vi "Parse Opening Tag.vi"(8 "Error In":errorcluster, 11 "Parser In":refnum<class "Parser.lvclass">) -> (0 "Error Out":errorcluster, 3 "Parser Out":refnum<class "Parser.lvclass">)   [LabVIEW 2017, in "Mustache.lvlib" / "Parser.lvclass"]
uses:
  Parser.lvclass
  Parser.lvclass/Parser.ctl
  Public/Controls/States.ctl
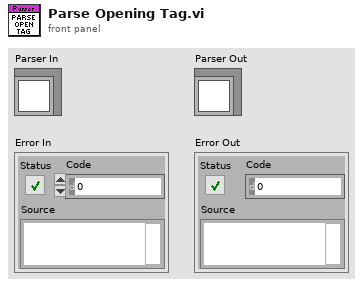
[diagram p1: front panel]
types:
  T1 = typedef "Mustache.lvlib/Parser.lvclass/States.ctl" = enum16{"Text", "Opening Tag", "Tag", "Closing Tag"}
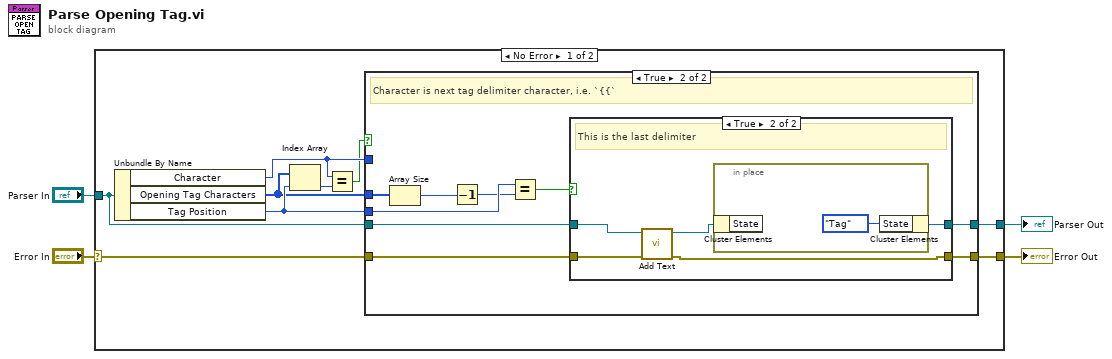
[diagram p0: block diagram]
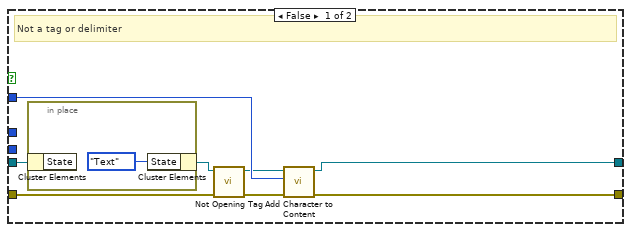
[diagram p2: hidden frame]
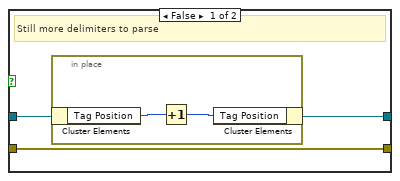
[diagram p3: hidden frame]
diagram:
  n1 = case shown="No Error" "Error In" {
    selector: "Error In" -> [w5 w43]
    tunnel: [w12 w43] -> w4
    tunnel: [w11 w44] -> w3
    tunnel: "Parser In" -> [w10 w44]
    frame No Error {
      n2 = Unbundle By Name(w10) -> ("Character"=w13:u8, "Opening Tag Characters"=w8:u8[], "Tag Position"=w9:i32)
      n3 = Index Array(array=w8, index=w9) -> (element=w6:u8)
      n4 = Equal?(x=w13, y=w6) -> (x = y?=w7:bool)
      n5 = case shown="True" w7 {
        tunnel: w8 -> [_ w31]
        tunnel: w9 -> [_ w29]
        tunnel: w5 -> [w14 w26]
        tunnel: w10 -> [w20 w25]
        tunnel: [w17 w24] -> w11
        tunnel: [w15 w23] -> w12
        tunnel: w13 -> [w21 _]
        frame False {
          # "Not a tag or delimiter"
          n6 = in-place {
            n7 = in-place-cluster #1(w20) -> ()  [unwired: 1 out]
            n8 = in-place-cluster #1("State"=States."Text") -> (w19:refnum<class "Parser.lvclass">)
          }
          n9 = call "Not Opening Tag.vi"("Error In"=w14, "Parser In"=w19) -> ("Error Out"=w16:errorcluster, "Parser Out"=w18:refnum<class "Parser.lvclass">)  [unwired: 8 in]
          n10 = call "Add Character to Content.vi"("Error In"=w16, "Character"=w21, "Parser In"=w18) -> ("Error Out"=w15:errorcluster, "Parser Out"=w17:refnum<class "Parser.lvclass">)  [unwired: 7 in]
        }
        frame True {
          # "Character is next tag delimiter character, i.e. `{{`"
          n11 = Array Size(array=w31) -> (size(s)=w30:i32)
          n12 = Decrement(x=w30) -> (x-1=w28:i32)
          n13 = Equal?(x=w29, y=w28) -> (x = y?=w27:bool)
          n14 = case shown="True" w27 {
            tunnel: w26 -> [w34 w38]
            tunnel: w25 -> [w33 w41]
            tunnel: [w32 w39] -> w24
            tunnel: [w34 w37] -> w23
            frame False {
              # "Still more delimiters to parse"
              n15 = in-place {
                n16 = in-place-cluster #2(w33) -> ("Tag Position"=w36:i32)
                n17 = Increment(x=w36) -> (x+1=w35:i32)
                n18 = in-place-cluster #2("Tag Position"=w35) -> (w32:refnum<class "Parser.lvclass">)
              }
            }
            frame True {
              # "This is the last delimiter"
              n19 = call "Add Text.vi"("Error In"=w38, "Parser In"=w41) -> ("Error Out"=w37:errorcluster, "Parser Out"=w40:refnum<class "Parser.lvclass">)  [unwired: 8 in]
              n20 = in-place {
                n21 = in-place-cluster #3(w40) -> ()  [unwired: 1 out]
                n22 = in-place-cluster #3("State"=States."Tag") -> (w39:refnum<class "Parser.lvclass">)
              }
            }
          }
        }
      }
    }
    frame Error {
    }
  }
  "Error Out" <- w4
  "Parser Out" <- w3
